vi "Get Serial Port.vi"(8 "error in (no error)":errorcluster, 11 "Serial Device in":refnum<class "Serial Device.lvclass">) -> (0 "error out":errorcluster, 2 "Serial Port":string, 3 "Serial Device out":refnum<class "Serial Device.lvclass">)   [LabVIEW 2017, in "Serial Device.lvclass"]
uses:
  Serial Device.lvclass
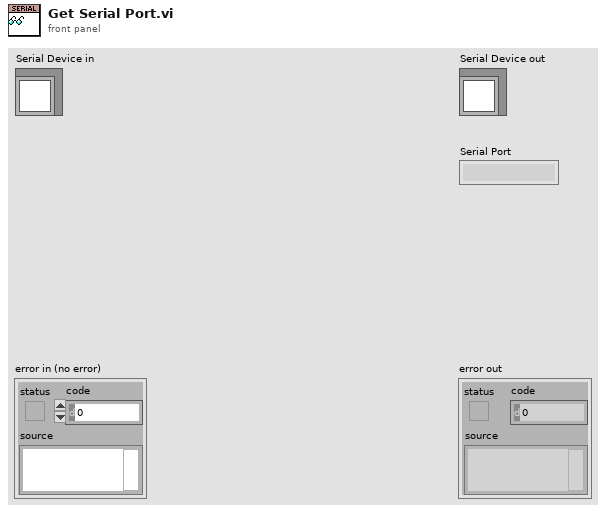
[diagram p1: front panel]
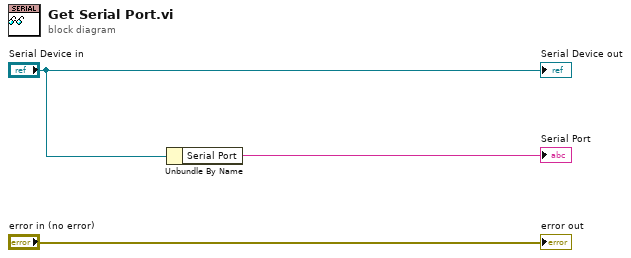
[diagram p0: block diagram]
diagram:
  n1 = Unbundle By Name("Serial Device in") -> ("Serial Port"=→"Serial Port":string)
  "error out" <- "error in (no error)"
  "Serial Device out" <- "Serial Device in"
